vi "App_Main Login.vi"(8 "error in":errorcluster) -> (0 "error out":errorcluster)   [LabVIEW 2018, in "Application 1.lvlib"]
uses:
  Application 1.lvlib
  Data Def/App_FGV Method.ctl
  Com VIs/Data Def/User Data.ctl
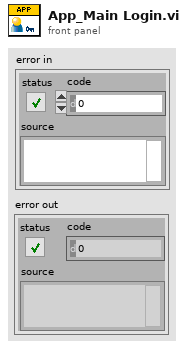
[diagram p1: front panel]
types:
  T1 = typedef "Application 1.lvlib/App_FGV Method.ctl" = enum16{"Get", "Put"}
  T2 = typedef "Application 1.lvlib/App_Configuration.ctl" = cluster{"Server IP":string, "User Name":string}
  T3 = typedef "Application 1.lvlib/App_Main Data.ctl" = cluster{"VI Refnum":refnum<vi>, "Subpanel":refnum<vi>, "Connection ID":refnum<k5>, "Meta data":T4[], "Main Queue":T6, "User Data":T7}
  T4 = typedef "stm_MetaElement.ctl" = cluster{"Name":T5}
  T5 = typedef "stm_MetaDataElement.ctl" = string
  T6 = typedef "Application 1.lvlib/App_Main Queue.ctl" = cluster{"Main Loop Queue":refnum<queue>}
  T7 = typedef "User Data.ctl" = cluster{"Name":string, "Email":string, "Phone Number":string, "User Picture":u32[][], "Last Login Time":timestamp}
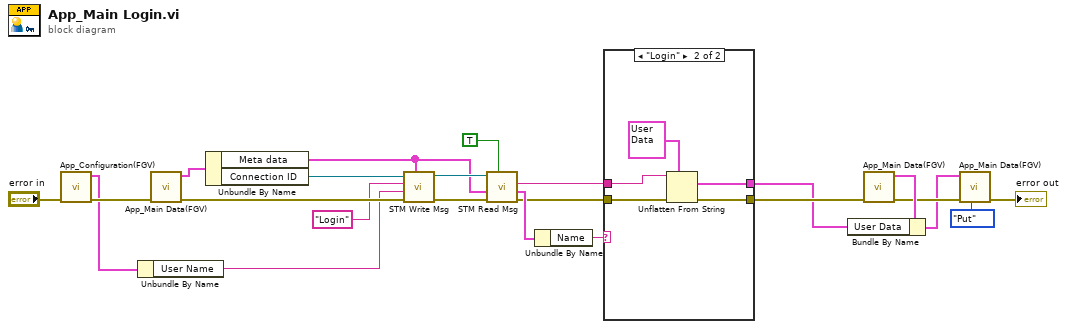
[diagram p0: block diagram]
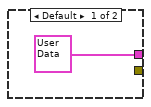
[diagram p2: hidden frame]
diagram:
  n1 = call "App_Configuration(FGV).vi"("error in"="error in") -> ("error out"=w4:errorcluster, "Configuration Out"=w3:T2)  [unwired: 9 in]
  n2 = Unbundle By Name(w3) -> ("User Name"=w2:string)
  n3 = call "App_Main Data(FGV).vi"("error in"=w4) -> ("error out"=w15:errorcluster, "Main Data Out"=w16:T3)  [unwired: 9 in]
  n4 = Unbundle By Name(w16) -> ("Meta data"=w10:T4[], "Connection ID"=w14:refnum<k5>)
  n5 = call "STM Write Msg.vi"("Meta data"=w10, "error in (no error)"=w15, "Data"=w2, "Name"="Login", "connection ID"=w14) -> ("error out"=w12:errorcluster, "connection ID out"=w11:refnum<k5>)  [unwired: 5 in]
  n6 = call "STM Read Msg.vi"("Ignore Timeout Error"=TRUE, "error in"=w12, "Meta data"=w10, "connection ID"=w11) -> ("error out"=w7:errorcluster, "Meta element"=w9:T4, "data string"=w6:string)  [unwired: 2 in, 3 out]
  n7 = Unbundle By Name(w9) -> ("Name"=w8:T5)
  n8 = case shown="\"Login\"" w8 {
    tunnel: w7 -> [_ w29]
    tunnel: w6 -> [_ w28]
    tunnel: [T7 {"Name"="Guest", "Email"="", "Phone Number"="", "User Picture"=array225x225[50625 elements], "Last Login Time"=timestamp(0 s since 1904-01-01)} ("User Data") w26] -> w21
    tunnel: [_ w25] -> w23
    frame Default {
    }
    frame "Login" {
      n9 = Unflatten From String(type=T7 {"Name"="", "Email"="", "Phone Number"="", "User Picture"=[], "Last Login Time"=timestamp(0 s since 1904-01-01)} ("User Data"), binary string=w28, error in (no error)=w29) -> (value=w26:T7, error out=w25:errorcluster)  [unwired: 2 in, 1 out]
    }
  }
  n10 = call "App_Main Data(FGV).vi"("error in"=w23) -> ("error out"=w20:errorcluster, "Main Data Out"=w22:T3)  [unwired: 9 in]
  n11 = Bundle By Name(cluster=w22, "User Data"=w21) -> (w19:T3)
  n12 = call "App_Main Data(FGV).vi"("FGV Method"=App_FGV_Method."Put", "error in"=w20, "Main Data In"=w19) -> ("error out"=→"error out":errorcluster)  [unwired: 7 in, 1 out]
